vi "Anritsu_MT8852B_YYLL_GetResult.vi"(8 "error in":errorcluster, 11 "VISA resource in":refnum<visa-resource-name>) -> (0 "error out":errorcluster, 1 "ValidString":string, 2 "Valid OK?":bool, 3 "VISA resource out":refnum<visa-resource-name>, 4 "Anritsu_MT8852B_YYLL_Result":T1={"AnritsuMT8852B_OP_Low_Avgpower"=-9999.0, "AnritsuMT8852B_OP_Low_Peakpower"=-9999.0, "AnritsuMT8852B_OP_Med_Avgpower"=-9999.0, "AnritsuMT8852B_OP_Med_Peakpower"=-9999.0, "AnritsuMT8852B_OP_Hig_Avgpower"=-9999.0, "AnritsuMT8852B_OP_Hig_Peakpower"=-9999.0, "AnritsuMT8852B_IC_Low_PositiveOffset"=-9999.0, "AnritsuMT8852B_IC_Low_NegativeOffset"=-9999.0, "AnritsuMT8852B_IC_Low_AvgOffset"=-9999.0, "AnritsuMT8852B_IC_Med_PositiveOffset"=-9999.0, "AnritsuMT8852B_IC_Med_NegativeOffset"=-9999.0, "AnritsuMT8852B_IC_Med_AvgOffset"=-9999.0, "AnritsuMT8852B_IC_Hig_PositiveOffset"=-9999.0, "AnritsuMT8852B_IC_Hig_NegativeOffset"=-9999.0, "AnritsuMT8852B_IC_Hig_AvgOffset"=-9999.0, "AnritsuMT8852B_SS_Low_BitErrorRate"=-9999.0, "AnritsuMT8852B_SS_Low_FrameErrorRate"=-9999.0, "AnritsuMT8852B_SS_Med_BitErrorRate"=-9999.0, "AnritsuMT8852B_SS_Med_FrameErrorRate"=-9999.0, "AnritsuMT8852B_SS_Hig_BitErrorRate"=-9999.0, "AnritsuMT8852B_SS_Hig_FrameErrorRate"=-9999.0, "StandardLim_OP_Avg[-6,20]"=FALSE, "StandardLim_OP_Peak[<23]"=FALSE, "StandardLim_IC_Offset[75KHz]"=FALSE, "StandardLim_SS_BitErrorRate[<0.1]"=FALSE, "StandardLim_SS_FrameErrorRate[<100]"=FALSE})   [LabVIEW 2017]
uses:
  Anritsu_MT8852B_YYLL_Result.ctl
  <vilib>/regexp/Match Regular Expression.xnode
panel:
  out "READ EUT ADDR":string
  in  "EUT ADDR Check & ReadedClear":bool
  # "TESTING>>>\nResult！！！"
  # "MT8852B"
  # "Anritsu"
  # "YYLL"
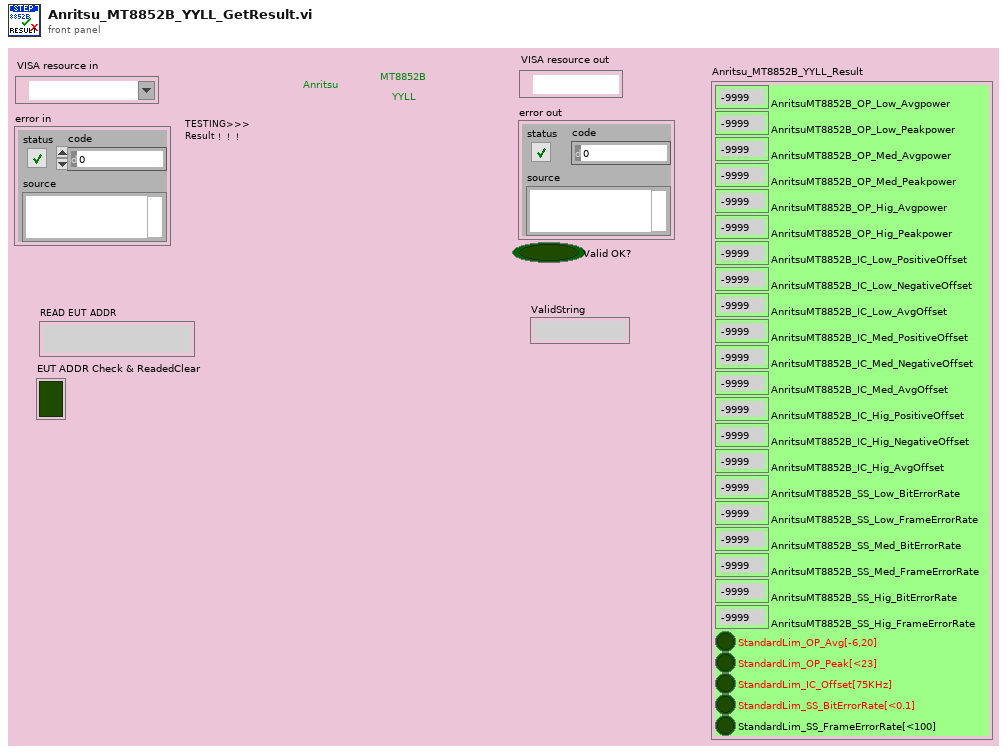
[diagram p1: front panel]
types:
  T1 = typedef "Anritsu_MT8852B_YYLL_Result.ctl" = cluster{"AnritsuMT8852B_OP_Low_Avgpower":dbl, "AnritsuMT8852B_OP_Low_Peakpower":dbl, "AnritsuMT8852B_OP_Med_Avgpower":dbl, "AnritsuMT8852B_OP_Med_Peakpower":dbl, "AnritsuMT8852B_OP_Hig_Avgpower":dbl, "AnritsuMT8852B_OP_Hig_Peakpower":dbl, "AnritsuMT8852B_IC_Low_PositiveOffset":dbl, "AnritsuMT8852B_IC_Low_NegativeOffset":dbl, "AnritsuMT8852B_IC_Low_AvgOffset":dbl, "AnritsuMT8852B_IC_Med_PositiveOffset":dbl, "AnritsuMT8852B_IC_Med_NegativeOffset":dbl, "AnritsuMT8852B_IC_Med_AvgOffset":dbl, "AnritsuMT8852B_IC_Hig_PositiveOffset":dbl, "AnritsuMT8852B_IC_Hig_NegativeOffset":dbl, "AnritsuMT8852B_IC_Hig_AvgOffset":dbl, "AnritsuMT8852B_SS_Low_BitErrorRate":dbl, "AnritsuMT8852B_SS_Low_FrameErrorRate":dbl, "AnritsuMT8852B_SS_Med_BitErrorRate":dbl, "AnritsuMT8852B_SS_Med_FrameErrorRate":dbl, "AnritsuMT8852B_SS_Hig_BitErrorRate":dbl, "AnritsuMT8852B_SS_Hig_FrameErrorRate":dbl, "StandardLim_OP_Avg[-6,20]":bool, "StandardLim_OP_Peak[<23]":bool, "StandardLim_IC_Offset[75KHz]":bool, "StandardLim_SS_BitErrorRate[<0.1]":bool, "StandardLim_SS_FrameErrorRate[<100]":bool}
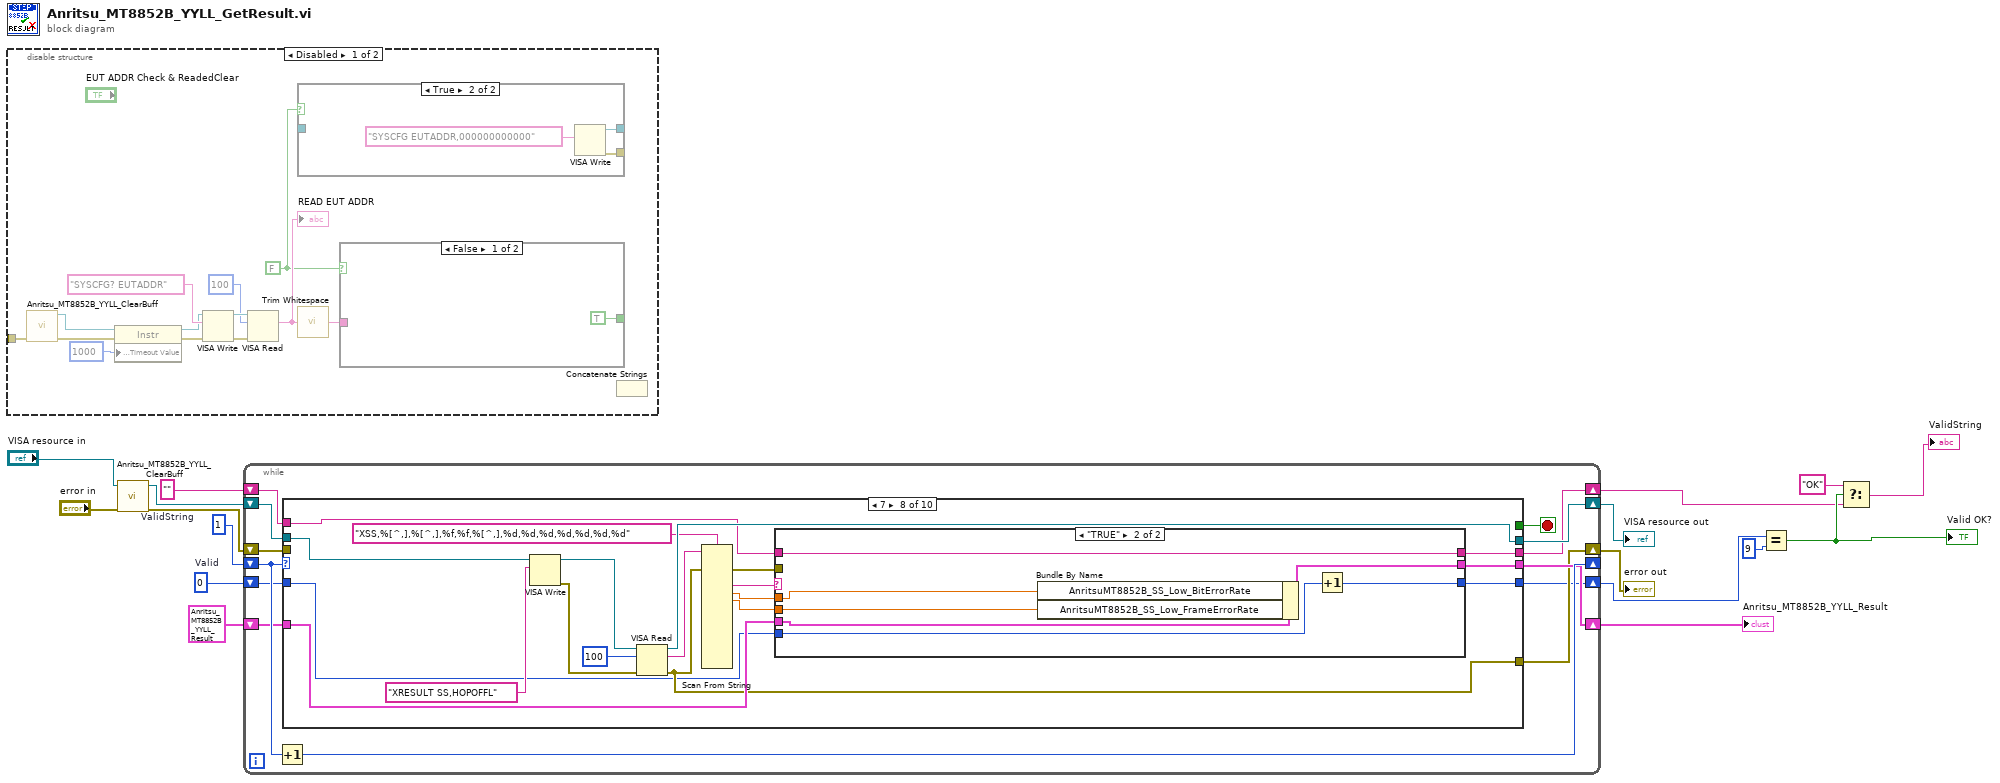
[diagram p0: block diagram]
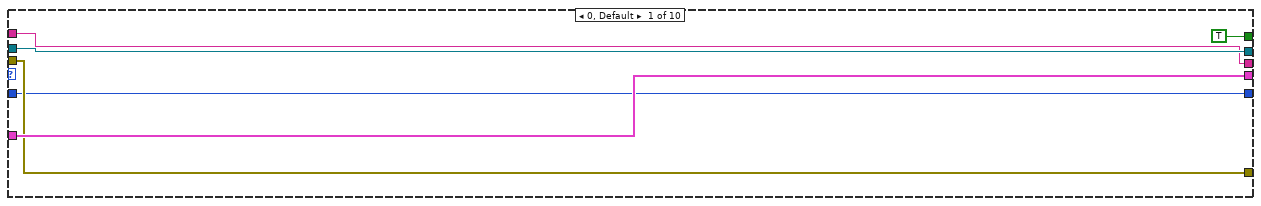
[diagram p2: hidden frame]
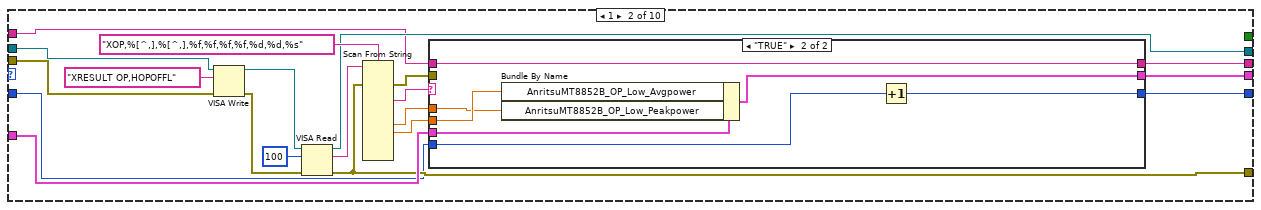
[diagram p3: hidden frame]
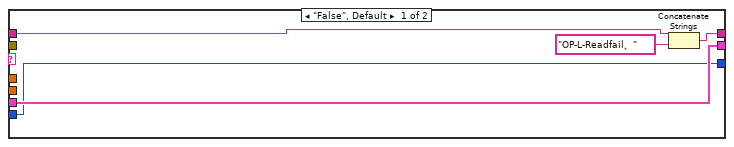
[diagram p4: hidden frame]
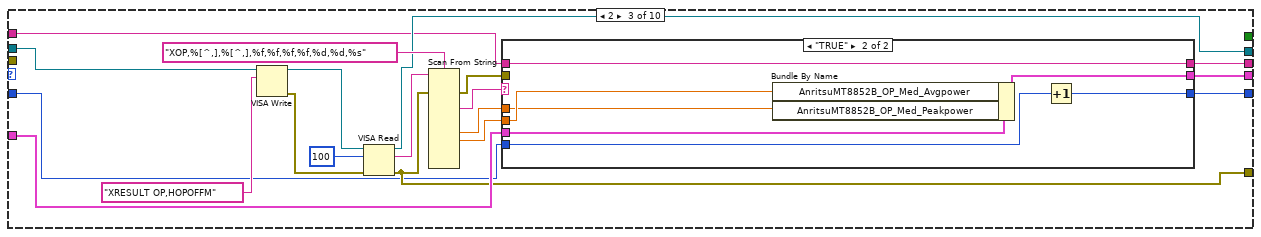
[diagram p5: hidden frame]
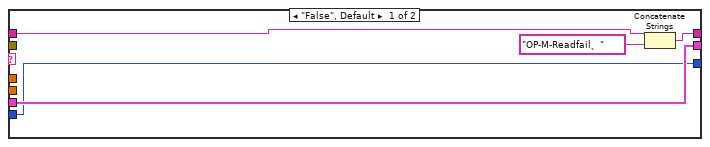
[diagram p6: hidden frame]
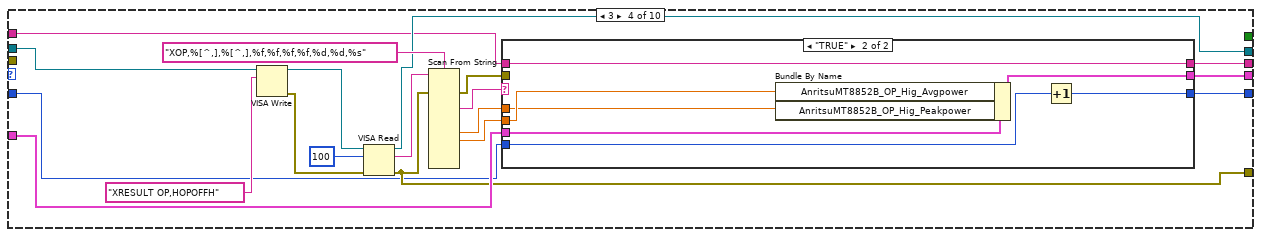
[diagram p7: hidden frame]
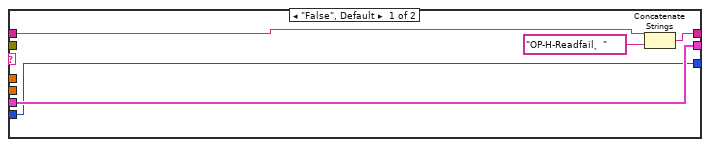
[diagram p8: hidden frame]
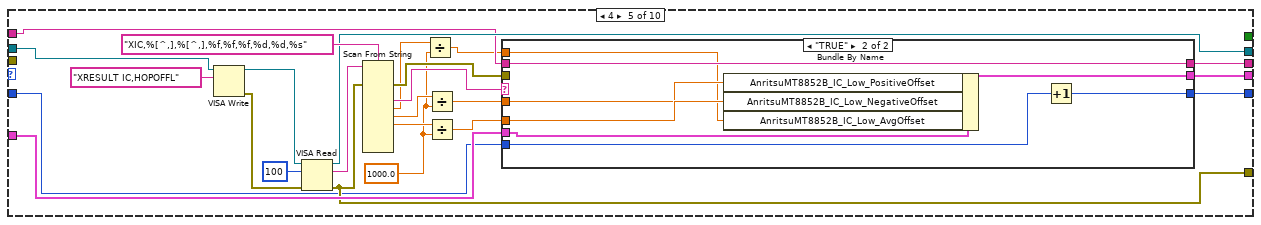
[diagram p9: hidden frame]
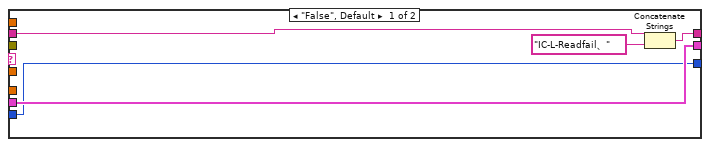
[diagram p10: hidden frame]
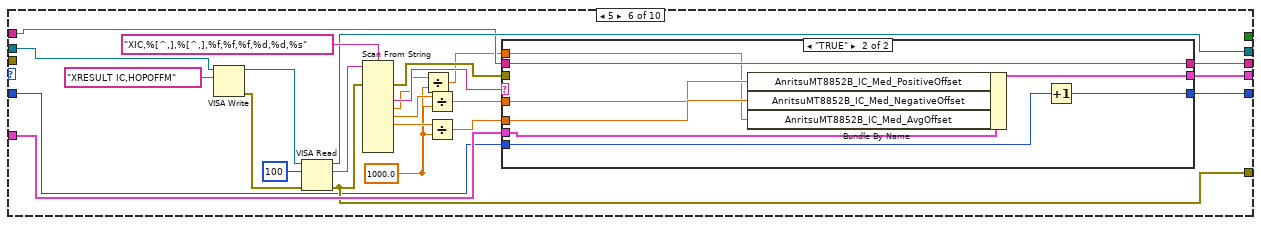
[diagram p11: hidden frame]
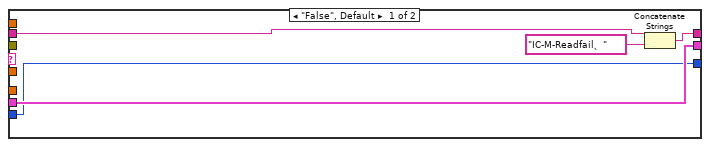
[diagram p12: hidden frame]
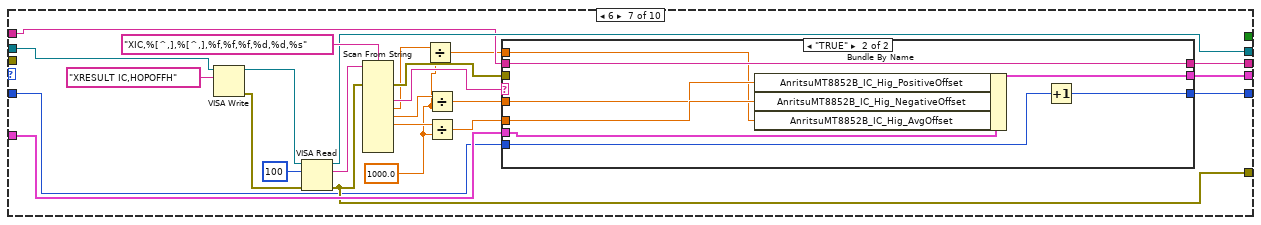
[diagram p13: hidden frame]
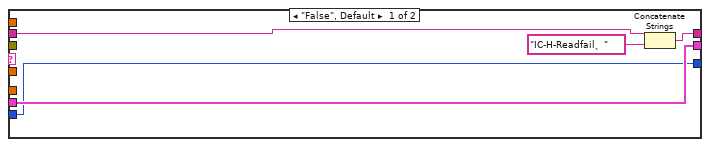
[diagram p14: hidden frame]
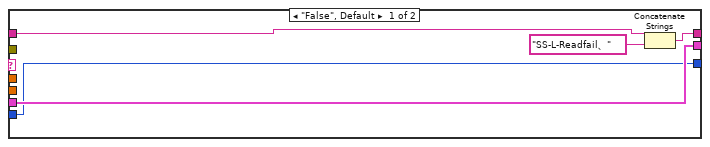
[diagram p15: hidden frame]
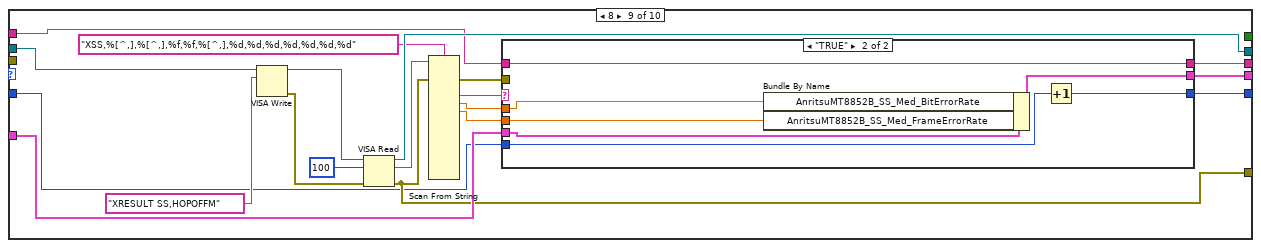
[diagram p16: hidden frame]
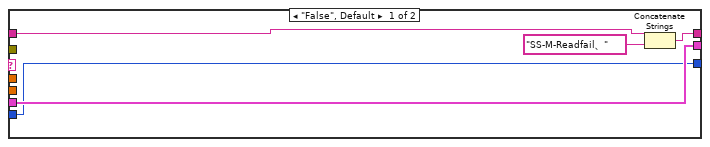
[diagram p17: hidden frame]
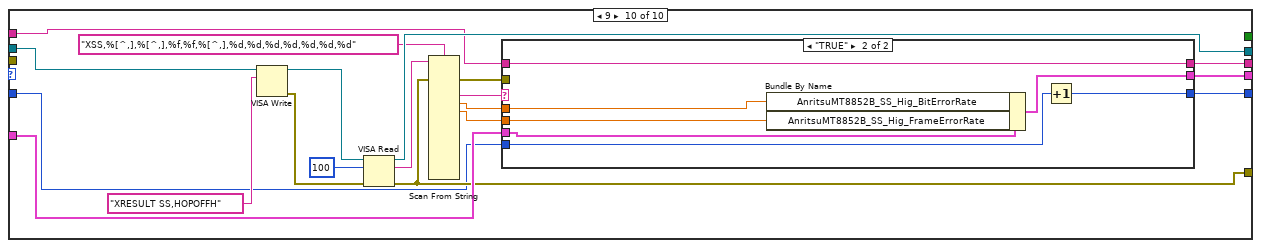
[diagram p18: hidden frame]
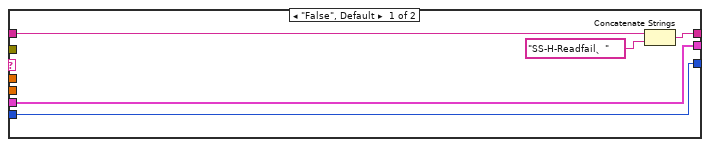
[diagram p19: hidden frame]
diagram:
  w5 = ""  # ValidString
  w8 = 0  # Valid
  n1 = disable-structure shown="Disabled" {
    disable-tunnel: _ -> [w19 _]
    frame Disabled {
      w18 = FALSE
      n2 = call "Anritsu_MT8852B_YYLL_ClearBuff.vi"("error IO"=w19) -> ("error IO 2"=w21:errorcluster, "VISA resource name 2"=w20:refnum<visa-resource-name>)  [unwired: 8 in, 1 out]
      n3 = property class="Instr"(reference=w20, error in=w21, "General Settings:Timeout Value"=u32 1000) -> (reference out=w25:refnum<visa-resource-name>, error out=w24:errorcluster)
      n4 = VISA Write(VISA resource name=w25, write buffer="SYSCFG? EUTADDR" ("write buffer (\"\")"), error in (no error)=w24) -> (VISA resource name out=w29:refnum<visa-resource-name>, error out=w26:errorcluster)  [unwired: 1 out]
      n5 = VISA Read(VISA resource name=w29, byte count=u32 100 ("byte count (0)"), error in (no error)=w26) -> (read buffer=w23:string)  [unwired: 3 out]
      "READ EUT ADDR" <- w23
      n6 = case shown="True" w18 {
        tunnel: [w31 w33] -> _
        tunnel: [_ w32] -> _
        tunnel: _ -> [w31 _]
        frame False {
        }
        frame True {
          n7 = VISA Write(write buffer="SYSCFG EUTADDR,000000000000" ("Substring")) -> (VISA resource name out=w33:refnum<visa-resource-name>, error out=w32:errorcluster)  [unwired: 2 in, 1 out]
        }
      }
      n8 = call <vilib>:"Trim Whitespace.vi"("string"=w23) -> ("trimmed string"=w22:string)  [unwired: 1 in]
      n9 = case shown="False" w18 {
        tunnel: w22 -> [_ w39]
        tunnel: [TRUE w36] -> _
        frame False {
        }
        frame True {
          n10 = Empty String/Path?(string/path=w39) -> (empty?=w41:bool)
          n11 = xnode "Match Regular Expression"("input string"=w39, "regular expression"="\\w{12}") -> ("whole match"=w42:string)  [unwired: 4 in, 4 out]
          n12 = Equal?(x=w39, y=w42) -> (x = y?=w40:bool)
          n13 = Not Equal?(x=w39, y="000000000000") -> (x != y?=w37:bool)
          n14 = Compound Arithmetic op=AND(w40, invert w41, w37) -> (w36:bool)
        }
      }
      n15 = Concatenate Strings() -> ()  [unwired: 2 in, 1 out]
    }
    frame Enabled {
    }
  }
  n16 = call "Anritsu_MT8852B_YYLL_ClearBuff.vi"("error IO"="error in", "VISA resource name"="VISA resource in") -> ("error IO 2"=w9:errorcluster, "VISA resource name 2"=w10:refnum<visa-resource-name>)  [unwired: 7 in, 1 out]
  n17 = while {
    shift-right: [w169] -> _
    shift-left: 1 -> [w170]
    shift-right: [w166] -> w15
    shift-left: w10 -> [w168]
    shift-right: [w165] -> w13
    shift-left: T1 {"AnritsuMT8852B_OP_Low_Avgpower"=-9999.0, "AnritsuMT8852B_OP_Low_Peakpower"=-9999.0, "AnritsuMT8852B_OP_Med_Avgpower"=-9999.0, "AnritsuMT8852B_OP_Med_Peakpower"=-9999.0, "AnritsuMT8852B_OP_Hig_Avgpower"=-9999.0, "AnritsuMT8852B_OP_Hig_Peakpower"=-9999.0, "AnritsuMT8852B_IC_Low_PositiveOffset"=-9999.0, "AnritsuMT8852B_IC_Low_NegativeOffset"=-9999.0, "AnritsuMT8852B_IC_Low_AvgOffset"=-9999.0, "AnritsuMT8852B_IC_Med_PositiveOffset"=-9999.0, "AnritsuMT8852B_IC_Med_NegativeOffset"=-9999.0, "AnritsuMT8852B_IC_Med_AvgOffset"=-9999.0, "AnritsuMT8852B_IC_Hig_PositiveOffset"=-9999.0, "AnritsuMT8852B_IC_Hig_NegativeOffset"=-9999.0, "AnritsuMT8852B_IC_Hig_AvgOffset"=-9999.0, "AnritsuMT8852B_SS_Low_BitErrorRate"=-9999.0, "AnritsuMT8852B_SS_Low_FrameErrorRate"=-9999.0, "AnritsuMT8852B_SS_Med_BitErrorRate"=-9999.0, "AnritsuMT8852B_SS_Med_FrameErrorRate"=-9999.0, "AnritsuMT8852B_SS_Hig_BitErrorRate"=-9999.0, "AnritsuMT8852B_SS_Hig_FrameErrorRate"=-9999.0, "StandardLim_OP_Avg[-6,20]"=FALSE, "StandardLim_OP_Peak[<23]"=FALSE, "StandardLim_IC_Offset[75KHz]"=FALSE, "StandardLim_SS_BitErrorRate[<0.1]"=FALSE, "StandardLim_SS_FrameErrorRate[<100]"=FALSE} ("Anritsu_MT8852B_YYLL_Result") -> [w164]
    shift-right: [w163] -> w14
    shift-left: w9 -> [w162]
    shift-right: [w161] -> w7
    shift-left: w8 -> [w160]
    shift-right: [w159] -> w3
    shift-left: w5 -> [w158]
    stop <- w167 stop-if-true
    n18 = Increment(x=w170) -> (x+1=w169:i32)
    n19 = case shown="7" w170 {
      tunnel: w168 -> [w175 w187 w218 w249 w287 w324 w361 w395 w426 w457]
      tunnel: [TRUE _ _ _ _ _ _ _ _ _] -> w167
      tunnel: [w175 w186 w217 w248 w286 w323 w360 w394 w425 w456] -> w166
      tunnel: [w174 w184 w215 w246 w284 w321 w358 w390 w421 w452] -> w165
      tunnel: w164 -> [w174 w185 w216 w247 w285 w322 w359 w391 w422 w453]
      tunnel: [w173 w181 w213 w244 w278 w315 w352 w386 w417 w448] -> w163
      tunnel: w162 -> [w173 w183 _ _ _ _ _ _ _ _]
      tunnel: [w172 w180 w212 w243 w276 w314 w351 w385 w416 w447] -> w161
      tunnel: w160 -> [w172 w179 w211 w240 w277 w313 w350 w384 w415 w446]
      tunnel: [w171 w178 w209 w241 w274 w311 w348 w382 w413 w444] -> w159
      tunnel: w158 -> [w171 w177 w210 w242 w275 w312 w349 w383 w414 w445]
      frame 0, Default {
      }
      frame 1 {
        n20 = VISA Write(VISA resource name=w187, write buffer="XRESULT OP,HOPOFFL" ("write buffer (\"\")"), error in (no error)=w183) -> (VISA resource name out=w193:refnum<visa-resource-name>, error out=w192:errorcluster)  [unwired: 1 out]
        n21 = VISA Read(VISA resource name=w193, byte count=u32 100 ("byte count (0)"), error in (no error)=w192) -> (VISA resource name out=w186:refnum<visa-resource-name>, read buffer=w191:string, error out=w181:errorcluster)  [unwired: 1 out]
        n22 = Scan From String(format string="XOP,%[^,],%[^,],%f,%f,%f,%f,%d,%d,%s" ("Format String"), input string=w191, error in=w181) -> (error out=w182:errorcluster, output 2=w194:string, output 5=w196:dbl, output 6=w195:dbl)  [unwired: 16 in, 2 out]
        n23 = case shown="\"TRUE\"" w194 {
          tunnel: [w201 w208] -> w184
          tunnel: w195 -> [_ w207]
          tunnel: w196 -> [_ w206]
          tunnel: w185 -> [w201 w205]
          tunnel: w182 -> [_ _]
          tunnel: [w200 w203] -> w180
          tunnel: w179 -> [w200 w204]
          tunnel: [w198 w202] -> w178
          tunnel: w177 -> [w199 w202]
          frame "False", Default {
            n24 = Concatenate Strings(w199, "OP-L-Readfail、" ("string")) -> (w198:string)
          }
          frame "TRUE" {
            n25 = Bundle By Name(cluster=w205, "AnritsuMT8852B_OP_Low_Avgpower"=w207, "AnritsuMT8852B_OP_Low_Peakpower"=w206) -> (w208:T1)
            n26 = Increment(x=w204) -> (x+1=w203:i32)
          }
        }
      }
      frame 2 {
        n27 = VISA Write(VISA resource name=w218, write buffer="XRESULT OP,HOPOFFM" ("write buffer (\"\")")) -> (VISA resource name out=w224:refnum<visa-resource-name>, error out=w223:errorcluster)  [unwired: 1 in, 1 out]
        n28 = VISA Read(VISA resource name=w224, byte count=u32 100 ("byte count (0)"), error in (no error)=w223) -> (VISA resource name out=w217:refnum<visa-resource-name>, read buffer=w222:string, error out=w213:errorcluster)  [unwired: 1 out]
        n29 = Scan From String(format string="XOP,%[^,],%[^,],%f,%f,%f,%f,%d,%d,%s" ("Format String"), input string=w222, error in=w213) -> (error out=w214:errorcluster, output 2=w225:string, output 5=w227:dbl, output 6=w226:dbl)  [unwired: 16 in, 2 out]
        n30 = case shown="\"TRUE\"" w225 {
          tunnel: [w232 w239] -> w215
          tunnel: w226 -> [_ w238]
          tunnel: w227 -> [_ w237]
          tunnel: w216 -> [w232 w236]
          tunnel: w214 -> [_ _]
          tunnel: [w231 w234] -> w212
          tunnel: w211 -> [w231 w235]
          tunnel: w210 -> [w229 w233]
          tunnel: [w228 w233] -> w209
          frame "False", Default {
            n31 = Concatenate Strings(w229, "OP-M-Readfail、" ("string")) -> (w228:string)
          }
          frame "TRUE" {
            n32 = Bundle By Name(cluster=w236, "AnritsuMT8852B_OP_Med_Avgpower"=w238, "AnritsuMT8852B_OP_Med_Peakpower"=w237) -> (w239:T1)
            n33 = Increment(x=w235) -> (x+1=w234:i32)
          }
        }
      }
      frame 3 {
        n34 = VISA Write(VISA resource name=w249, write buffer="XRESULT OP,HOPOFFH" ("write buffer (\"\")")) -> (VISA resource name out=w255:refnum<visa-resource-name>, error out=w254:errorcluster)  [unwired: 1 in, 1 out]
        n35 = VISA Read(VISA resource name=w255, byte count=u32 100 ("byte count (0)"), error in (no error)=w254) -> (VISA resource name out=w248:refnum<visa-resource-name>, read buffer=w253:string, error out=w244:errorcluster)  [unwired: 1 out]
        n36 = Scan From String(format string="XOP,%[^,],%[^,],%f,%f,%f,%f,%d,%d,%s" ("Format String"), input string=w253, error in=w244) -> (error out=w245:errorcluster, output 2=w256:string, output 5=w258:dbl, output 6=w257:dbl)  [unwired: 16 in, 2 out]
        n37 = case shown="\"TRUE\"" w256 {
          tunnel: [w263 w270] -> w246
          tunnel: w257 -> [_ w269]
          tunnel: w258 -> [_ w268]
          tunnel: w247 -> [w263 w267]
          tunnel: w245 -> [_ _]
          tunnel: [w262 w265] -> w243
          tunnel: w240 -> [w262 w266]
          tunnel: w242 -> [w260 w264]
          tunnel: [w259 w264] -> w241
          frame "False", Default {
            n38 = Concatenate Strings(w260, "OP-H-Readfail、" ("string")) -> (w259:string)
          }
          frame "TRUE" {
            n39 = Bundle By Name(cluster=w267, "AnritsuMT8852B_OP_Hig_Avgpower"=w269, "AnritsuMT8852B_OP_Hig_Peakpower"=w268) -> (w270:T1)
            n40 = Increment(x=w266) -> (x+1=w265:i32)
          }
        }
      }
      frame 4 {
        w272 = 1000.0 ("x")
        n41 = VISA Write(VISA resource name=w287, write buffer="XRESULT IC,HOPOFFL" ("write buffer (\"\")")) -> (VISA resource name out=w293:refnum<visa-resource-name>, error out=w292:errorcluster)  [unwired: 1 in, 1 out]
        n42 = VISA Read(VISA resource name=w293, byte count=u32 100 ("byte count (0)"), error in (no error)=w292) -> (VISA resource name out=w286:refnum<visa-resource-name>, read buffer=w291:string, error out=w278:errorcluster)  [unwired: 1 out]
        n43 = Scan From String(format string="XIC,%[^,],%[^,],%f,%f,%f,%d,%d,%s" ("Format String"), input string=w291, error in=w278) -> (error out=w279:errorcluster, output 2=w294:string, output 3=w273:dbl, output 4=w283:dbl, output 5=w281:dbl)  [unwired: 13 in, 2 out]
        n44 = Divide(x=w273, y=w272) -> (x/y=w271:dbl)
        n45 = Divide(x=w283, y=w272) -> (x/y=w282:dbl)
        n46 = Divide(x=w281, y=w272) -> (x/y=w280:dbl)
        n47 = case shown="\"TRUE\"" w294 {
          tunnel: [w299 w307] -> w284
          tunnel: w285 -> [w299 w306]
          tunnel: w280 -> [_ w305]
          tunnel: w282 -> [_ w304]
          tunnel: w279 -> [_ _]
          tunnel: w277 -> [w298 w303]
          tunnel: [w298 w302] -> w276
          tunnel: w275 -> [w296 w301]
          tunnel: [w295 w301] -> w274
          tunnel: w271 -> [_ w300]
          frame "False", Default {
            n48 = Concatenate Strings(w296, "IC-L-Readfail、" ("string")) -> (w295:string)
          }
          frame "TRUE" {
            n49 = Bundle By Name(cluster=w306, "AnritsuMT8852B_IC_Low_PositiveOffset"=w304, "AnritsuMT8852B_IC_Low_NegativeOffset"=w305, "AnritsuMT8852B_IC_Low_AvgOffset"=w300) -> (w307:T1)
            n50 = Increment(x=w303) -> (x+1=w302:i32)
          }
        }
      }
      frame 5 {
        w309 = 1000.0 ("x")
        n51 = VISA Write(VISA resource name=w324, write buffer="XRESULT IC,HOPOFFM" ("write buffer (\"\")")) -> (VISA resource name out=w330:refnum<visa-resource-name>, error out=w329:errorcluster)  [unwired: 1 in, 1 out]
        n52 = VISA Read(VISA resource name=w330, byte count=u32 100 ("byte count (0)"), error in (no error)=w329) -> (VISA resource name out=w323:refnum<visa-resource-name>, read buffer=w328:string, error out=w315:errorcluster)  [unwired: 1 out]
        n53 = Scan From String(format string="XIC,%[^,],%[^,],%f,%f,%f,%d,%d,%s" ("Format String"), input string=w328, error in=w315) -> (error out=w316:errorcluster, output 2=w331:string, output 3=w310:dbl, output 4=w320:dbl, output 5=w318:dbl)  [unwired: 13 in, 2 out]
        n54 = Divide(x=w310, y=w309) -> (x/y=w308:dbl)
        n55 = Divide(x=w320, y=w309) -> (x/y=w319:dbl)
        n56 = Divide(x=w318, y=w309) -> (x/y=w317:dbl)
        n57 = case shown="\"TRUE\"" w331 {
          tunnel: [w336 w344] -> w321
          tunnel: w322 -> [w336 w343]
          tunnel: w317 -> [_ w342]
          tunnel: w319 -> [_ w341]
          tunnel: w316 -> [_ _]
          tunnel: [w335 w339] -> w314
          tunnel: w313 -> [w335 w340]
          tunnel: w312 -> [w333 w338]
          tunnel: [w332 w338] -> w311
          tunnel: w308 -> [_ w337]
          frame "False", Default {
            n58 = Concatenate Strings(w333, "IC-M-Readfail、" ("string")) -> (w332:string)
          }
          frame "TRUE" {
            n59 = Bundle By Name(cluster=w343, "AnritsuMT8852B_IC_Med_PositiveOffset"=w341, "AnritsuMT8852B_IC_Med_NegativeOffset"=w342, "AnritsuMT8852B_IC_Med_AvgOffset"=w337) -> (w344:T1)
            n60 = Increment(x=w340) -> (x+1=w339:i32)
          }
        }
      }
      frame 6 {
        w346 = 1000.0 ("x")
        n61 = VISA Write(VISA resource name=w361, write buffer="XRESULT IC,HOPOFFH" ("write buffer (\"\")")) -> (VISA resource name out=w367:refnum<visa-resource-name>, error out=w366:errorcluster)  [unwired: 1 in, 1 out]
        n62 = VISA Read(VISA resource name=w367, byte count=u32 100 ("byte count (0)"), error in (no error)=w366) -> (VISA resource name out=w360:refnum<visa-resource-name>, read buffer=w365:string, error out=w352:errorcluster)  [unwired: 1 out]
        n63 = Scan From String(format string="XIC,%[^,],%[^,],%f,%f,%f,%d,%d,%s" ("Format String"), input string=w365, error in=w352) -> (error out=w353:errorcluster, output 2=w368:string, output 3=w347:dbl, output 4=w357:dbl, output 5=w355:dbl)  [unwired: 13 in, 2 out]
        n64 = Divide(x=w347, y=w346) -> (x/y=w345:dbl)
        n65 = Divide(x=w357, y=w346) -> (x/y=w356:dbl)
        n66 = Divide(x=w355, y=w346) -> (x/y=w354:dbl)
        n67 = case shown="\"TRUE\"" w368 {
          tunnel: [w373 w381] -> w358
          tunnel: w359 -> [w373 w380]
          tunnel: w354 -> [_ w379]
          tunnel: w356 -> [_ w378]
          tunnel: w353 -> [_ _]
          tunnel: [w372 w376] -> w351
          tunnel: w350 -> [w372 w377]
          tunnel: w349 -> [w370 w375]
          tunnel: [w369 w375] -> w348
          tunnel: w345 -> [_ w374]
          frame "False", Default {
            n68 = Concatenate Strings(w370, "IC-H-Readfail、" ("string")) -> (w369:string)
          }
          frame "TRUE" {
            n69 = Bundle By Name(cluster=w380, "AnritsuMT8852B_IC_Hig_PositiveOffset"=w378, "AnritsuMT8852B_IC_Hig_NegativeOffset"=w379, "AnritsuMT8852B_IC_Hig_AvgOffset"=w374) -> (w381:T1)
            n70 = Increment(x=w377) -> (x+1=w376:i32)
          }
        }
      }
      frame 7 {
        n71 = VISA Write(VISA resource name=w395, write buffer="XRESULT SS,HOPOFFL" ("write buffer (\"\")")) -> (VISA resource name out=w400:refnum<visa-resource-name>, error out=w399:errorcluster)  [unwired: 1 in, 1 out]
        n72 = VISA Read(VISA resource name=w400, byte count=u32 100 ("byte count (0)"), error in (no error)=w399) -> (VISA resource name out=w394:refnum<visa-resource-name>, read buffer=w397:string, error out=w386:errorcluster)  [unwired: 1 out]
        n73 = Scan From String(format string="XSS,%[^,],%[^,],%f,%f,%[^,],%d,%d,%d,%d,%d,%d,%d" ("Format String"), input string=w397, error in=w386) -> (error out=w387:errorcluster, output 2=w392:string, output 3=w389:dbl, output 4=w388:dbl)  [unwired: 22 in, 2 out]
        n74 = case shown="\"TRUE\"" w392 {
          tunnel: [w405 w412] -> w390
          tunnel: w391 -> [w405 w411]
          tunnel: w389 -> [_ w410]
          tunnel: w388 -> [_ w409]
          tunnel: w387 -> [_ _]
          tunnel: [w404 w407] -> w385
          tunnel: w384 -> [w404 w408]
          tunnel: w383 -> [w402 w406]
          tunnel: [w401 w406] -> w382
          frame "False", Default {
            n75 = Concatenate Strings(w402, "SS-L-Readfail、" ("string")) -> (w401:string)
          }
          frame "TRUE" {
            n76 = Bundle By Name(cluster=w411, "AnritsuMT8852B_SS_Low_BitErrorRate"=w410, "AnritsuMT8852B_SS_Low_FrameErrorRate"=w409) -> (w412:T1)
            n77 = Increment(x=w408) -> (x+1=w407:i32)
          }
        }
      }
      frame 8 {
        n78 = VISA Write(VISA resource name=w426, write buffer="XRESULT SS,HOPOFFM" ("write buffer (\"\")")) -> (VISA resource name out=w431:refnum<visa-resource-name>, error out=w430:errorcluster)  [unwired: 1 in, 1 out]
        n79 = VISA Read(VISA resource name=w431, byte count=u32 100 ("byte count (0)"), error in (no error)=w430) -> (VISA resource name out=w425:refnum<visa-resource-name>, read buffer=w428:string, error out=w417:errorcluster)  [unwired: 1 out]
        n80 = Scan From String(format string="XSS,%[^,],%[^,],%f,%f,%[^,],%d,%d,%d,%d,%d,%d,%d" ("Format String"), input string=w428, error in=w417) -> (error out=w418:errorcluster, output 2=w423:string, output 3=w420:dbl, output 4=w419:dbl)  [unwired: 22 in, 2 out]
        n81 = case shown="\"TRUE\"" w423 {
          tunnel: [w436 w443] -> w421
          tunnel: w422 -> [w436 w442]
          tunnel: w420 -> [_ w441]
          tunnel: w419 -> [_ w440]
          tunnel: w418 -> [_ _]
          tunnel: [w435 w438] -> w416
          tunnel: w415 -> [w435 w439]
          tunnel: w414 -> [w433 w437]
          tunnel: [w432 w437] -> w413
          frame "False", Default {
            n82 = Concatenate Strings(w433, "SS-M-Readfail、" ("string")) -> (w432:string)
          }
          frame "TRUE" {
            n83 = Bundle By Name(cluster=w442, "AnritsuMT8852B_SS_Med_BitErrorRate"=w441, "AnritsuMT8852B_SS_Med_FrameErrorRate"=w440) -> (w443:T1)
            n84 = Increment(x=w439) -> (x+1=w438:i32)
          }
        }
      }
      frame 9 {
        n85 = VISA Write(VISA resource name=w457, write buffer="XRESULT SS,HOPOFFH" ("write buffer (\"\")")) -> (VISA resource name out=w462:refnum<visa-resource-name>, error out=w461:errorcluster)  [unwired: 1 in, 1 out]
        n86 = VISA Read(VISA resource name=w462, byte count=u32 100 ("byte count (0)"), error in (no error)=w461) -> (VISA resource name out=w456:refnum<visa-resource-name>, read buffer=w459:string, error out=w448:errorcluster)  [unwired: 1 out]
        n87 = Scan From String(format string="XSS,%[^,],%[^,],%f,%f,%[^,],%d,%d,%d,%d,%d,%d,%d" ("Format String"), input string=w459, error in=w448) -> (error out=w449:errorcluster, output 2=w454:string, output 3=w451:dbl, output 4=w450:dbl)  [unwired: 22 in, 2 out]
        n88 = case shown="\"TRUE\"" w454 {
          tunnel: [w467 w474] -> w452
          tunnel: w453 -> [w467 w473]
          tunnel: w451 -> [_ w472]
          tunnel: w450 -> [_ w471]
          tunnel: w449 -> [_ _]
          tunnel: [w466 w469] -> w447
          tunnel: w446 -> [w466 w470]
          tunnel: w445 -> [w464 w468]
          tunnel: [w463 w468] -> w444
          frame "False", Default {
            n89 = Concatenate Strings(w464, "SS-H-Readfail、" ("string")) -> (w463:string)
          }
          frame "TRUE" {
            n90 = Bundle By Name(cluster=w473, "AnritsuMT8852B_SS_Hig_BitErrorRate"=w472, "AnritsuMT8852B_SS_Hig_FrameErrorRate"=w471) -> (w474:T1)
            n91 = Increment(x=w470) -> (x+1=w469:i32)
          }
        }
      }
    }
  }
  "VISA resource out" <- w15
  "error out" <- w14
  "Anritsu_MT8852B_YYLL_Result" <- w13
  n92 = Equal?(x=w7, y=9) -> (x = y?=w4:bool)
  "Valid OK?" <- w4
  n93 = Select(t="OK", s=w4, f=w3) -> (s? t:f=→"ValidString":string)
